vi "Hatch Intake.vi"(0 "Turn On?":bool, 1 "Close Ref":string, 2 "Drive Ref":string) -> ()   [LabVIEW 2018]
uses:
  <vilib>/Rock Robotics/WPI/Solenoid/WPI_SolenoidValue.ctl
  <vilib>/Rock Robotics/WPI/Utilities/WPI_GetSetVariantRefNum.vi
  <vilib>/Rock Robotics/Network Tables/NT Read Number.vi
  <vilib>/Rock Robotics/WPI/RobotDrive/WPI_RobotDriveArcadeDrive_Standard(NoSaturation).vi
  <vilib>/Rock Robotics/WPI/Solenoid/WPI_SolenoidSetEnum.vi
  Robot Global Data.vi
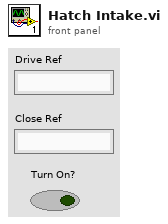
[diagram p1: front panel]
types:
  T1 = typedef "WPI_SolenoidValue.ctl" = enum16{"Off", "On", "Forward", "Reverse"}
  T2 = typedef "WPI_SolenoidDevRef.ctl" = cluster{"DevStatus":errorcluster, "Pneumatics Control Module":u8, "Forward Solenoid Channel":T3, "Reverse Solenoid Channel":T3}
  T3 = typedef "WPI_SolenoidChannel.ctl" = enum8{"Solenoid 0", "Solenoid 1", "Solenoid 2", "Solenoid 3", "Solenoid 4", "Solenoid 5", "Solenoid 6", "Solenoid 7", "Invalid"}
  T4 = typedef "WPI_JoystickDevRef.ctl" = cluster{"Device":T5}
  T5 = typedef "WPI_JoystickDeviceEnum.ctl" = enum16{"USB 0", "USB 1", "USB 2", "USB 3", "USB 4", "USB 5"}
  T6 = typedef "WPI_RobotDriveDevRef.ctl" = cluster{"DevStatus":errorcluster, "Motors[]":T7[], "Square Inputs":bool, "Max Output":dbl}
  T7 = typedef "WPI_MotorControlDeviceRef.ctl" = cluster{"DeviceStatus":errorcluster, "Type":T8, "PWM":cluster{"PWM Channel":T9, "DeadBand":T10}, "CAN":cluster{"Device Number":u8, "SetOutput VI Ref":variant, "GetOutput VI Ref":variant, "Enable VI Ref":variant, "Disable VI Ref":variant, "Data":variant}, "Invert":bool, "DIO PWM":cluster{"PWM \"Enable\" Channel":T9, "DIOChannel":T11, "PWM Rate":dbl}}
  T8 = typedef "WPI_MotorControlType.ctl" = enum16{"PWM", "CAN", "DIO PWM"}
  T9 = typedef "FPGA_DIOPWMChannel.ctl" = enum8{"PWM 0", "PWM 1", "PWM 2", "PWM 3", "PWM 4", "PWM 5", "PWM 6", "PWM 7", "PWM 8", "PWM 9", "PWM MXP 0", "PWM MXP 1", "PWM MXP 2", "PWM MXP 3", "PWM MXP 4", "PWM MXP 5", "PWM MXP 6", "PWM MXP 7", "PWM MXP 8", "PWM MXP 9", "Invalid"}
  T10 = typedef "WPI_PWMDeadband.ctl" = cluster{"Name":string, "maxPositivePwm":i32, "minPositivePwm":i32, "centerPwm":i32, "maxNegativePwm":i32, "minNegativePwm":i32, "angularRange":u16}
  T11 = typedef "FPGA_DIOChannel.ctl" = enum8{"DIO 0", "DIO 1", "DIO 2", "DIO 3", "DIO 4", "DIO 5", "DIO 6", "DIO 7", "DIO 8", "DIO 9", "DIO MXP 0", "DIO MXP 1", "DIO MXP 2", "DIO MXP 3", "DIO MXP 4", "DIO MXP 5", "DIO MXP 6", "DIO MXP 7", "DIO MXP 8", "DIO MXP 9", "DIO MXP 10", "DIO MXP 11", "DIO MXP 12", "DIO MXP 13", "DIO MXP 14", "DIO MXP 15", "SPI Port CS1", "SPI Port CS2", "SPI Port CS3", "SPI Port MISO", "SPI Port MOSI", "Invalid"}
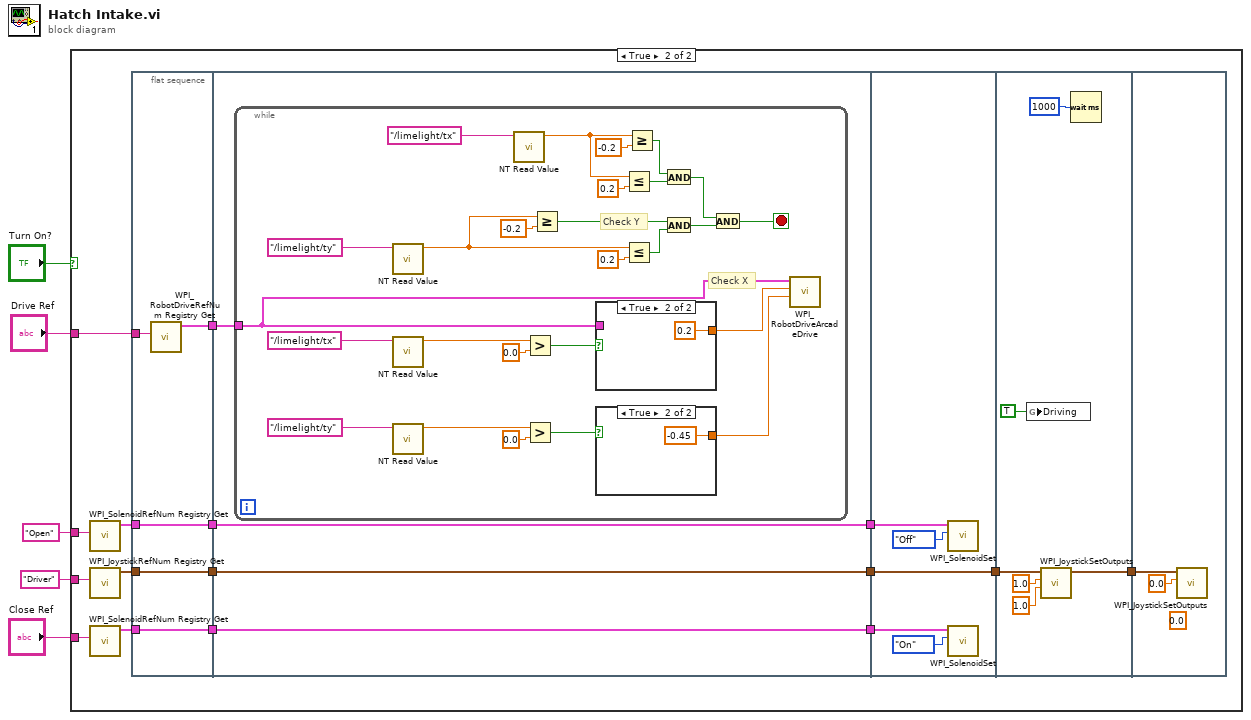
[diagram p0: block diagram]
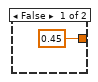
[diagram p3: hidden frame]
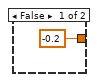
[diagram p4: hidden frame]
diagram:
  n1 = case shown="True" "Turn On?" {
    tunnel: "Close Ref" -> [_ w20]
    tunnel: "Drive Ref" -> [_ w21]
    tunnel: "Open" -> [_ w18]
    tunnel: "Driver" -> [_ w11]
    frame False {
    }
    frame True {
      n2 = call <vilib>:"WPI_SolenoidRefNum Registry Get.vi"("refnum name"=w18) -> ("SolenoidDevRef"=w12:T2)  [unwired: 9 in, 1 out]
      n3 = call <vilib>:"WPI_JoystickRefNum Registry Get.vi"("refnum name"=w11) -> ("JoystickDevRef"=w7:T4)  [unwired: 9 in, 1 out]
      n4 = call <vilib>:"WPI_SolenoidRefNum Registry Get.vi"("refnum name"=w20) -> ("SolenoidDevRef"=w15:T2)  [unwired: 9 in, 1 out]
      n5 = flat-sequence {
        tunnel: w21 -> [w26]
        tunnel: [w25] -> w19
        tunnel: [w24] -> w16
        tunnel: w15 -> [w24]
        tunnel: [w23] -> w13
        tunnel: w12 -> [w23]
        tunnel: [w22] -> w8
        tunnel: w7 -> [w22]
        tunnel: w19 -> [w30]
        tunnel: [w29] -> w17
        tunnel: w16 -> [w29]
        tunnel: [w28] -> w14
        tunnel: w13 -> [w28]
        tunnel: [w27] -> w9
        tunnel: w8 -> [w27]
        tunnel: w17 -> [w65]
        tunnel: w14 -> [w64]
        tunnel: [w61] -> w10
        tunnel: w9 -> [w61]
        tunnel: w10 -> [w71]
        tunnel: [w67] -> w6
        tunnel: w6 -> [w72]
        frame #0 {
          n6 = call <vilib>:"WPI_RobotDriveRefNum Registry Get.vi"("refnum name"=w26) -> ("RobotDriveDevRef"=w25:T6)  [unwired: 9 in, 1 out]
        }
        frame #1 {
          n7 = while {
            tunnel: w30 -> [w37]
            stop <- w46 stop-if-true
            # "Check Y"
            # "Check X"
            n8 = call-poly <vilib>:"NT Read Value.vi"("Name"="/limelight/ty") -> ("Numeric"=w42:dbl)  [unwired: 9 in, 1 out]
            n9 = call-poly <vilib>:"NT Read Value.vi"("Name"="/limelight/tx") -> ("Numeric"=w39:dbl)  [unwired: 9 in, 1 out]
            n10 = call-poly <vilib>:"NT Read Value.vi"("Name"="/limelight/ty") -> ("Numeric"=w35:dbl)  [unwired: 9 in, 1 out]
            n11 = call-poly <vilib>:"NT Read Value.vi"("Name"="/limelight/tx") -> ("Numeric"=w44:dbl)  [unwired: 9 in, 1 out]
            n12 = Greater?(x=w39, y=0.0) -> (0:w41:bool)
            n13 = Greater?(x=w35, y=0.0) -> (0:w33:bool)
            n14 = Greater Or Equal?(x=w42, y=-0.2) -> (x >= y?=w56:bool)
            n15 = case shown="True" w41 {
              tunnel: w37 -> [_ _]
              tunnel: [-0.2 0.2] -> w31
              frame False {
              }
              frame True {
              }
            }
            n16 = case shown="True" w33 {
              tunnel: [0.45 -0.45] -> w32
              frame False {
              }
              frame True {
              }
            }
            n17 = Less Or Equal?(x=w44, y=0.2) -> (x <= y?=w50:bool)
            n18 = Less Or Equal?(x=w42, y=0.2) -> (x <= y?=w55:bool)
            n19 = Greater Or Equal?(x=w44, y=-0.2) -> (x >= y?=w49:bool)
            n20 = And(x=w49, y=w50) -> (x .and. y?=w48:bool)
            n21 = And(x=w56, y=w55) -> (x .and. y?=w47:bool)
            n22 = And(x=w48, y=w47) -> (x .and. y?=w46:bool)
            n23 = call-poly <vilib>:"WPI_RobotDriveArcadeDrive.vi"("Y axis value"=w32, "X axis value"=w31, "RobotDriveDevRef"=w37) -> ()  [unwired: 6 in, 3 out]
          }
        }
        frame #2 {
          n24 = call-poly <vilib>:"WPI_SolenoidSet.vi"("Value"=WPI_SolenoidValue."Off", "SolenoidDevRef"=w64) -> ()  [unwired: 8 in, 2 out]
          n25 = call-poly <vilib>:"WPI_SolenoidSet.vi"("Value"=WPI_SolenoidValue."On", "SolenoidDevRef"=w65) -> ()  [unwired: 8 in, 2 out]
        }
        frame #3 {
          n26 = global write "Robot Global Data.vi" "Driving"(TRUE) -> ()
          n27 = call <vilib>:"WPI_JoystickSetOutputs.vi"("Right Rumble"=sgl 1.0, "Left Rumble"=sgl 1.0, "JoystickDevRef"=w71) -> ("JoystickDevRef"=w67:T4)  [unwired: 7 in, 1 out]
          n28 = Wait (ms)(milliseconds to wait=u32 1000) -> ()  [unwired: 1 out]
        }
        frame #4 {
          (unwired) sgl 0.0 ("Right Rumble")
          n29 = call <vilib>:"WPI_JoystickSetOutputs.vi"("Left Rumble"=sgl 0.0, "JoystickDevRef"=w72) -> ()  [unwired: 8 in, 2 out]
        }
      }
    }
  }
